vi "Start Call to results window.vi"(8 "Find Broadcast?":bool, 9 "Request VI Callers":refnum<vi>[](array[refnum]), 10 "Event":refnum<vi>) -> ()   [LabVIEW 2020, in "Panther Dashboard.lvlib"]
uses:
  Panther Dashboard.lvlib
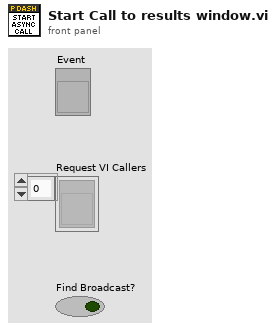
[diagram p1: front panel]
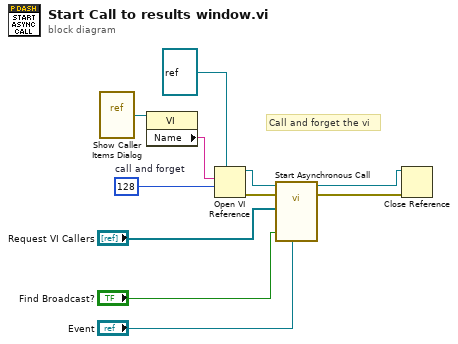
[diagram p0: block diagram]
diagram:
  w8 = 128  # call and forget
  # "Call and forget the vi"
  n1 = vi-ref "Show Caller Items Dialog.vi"() -> (w5:refnum<vi>)
  n2 = property class="VI"(reference=w5) -> ("Name"=w6:string)  [unwired: 1 in, 2 out]
  n3 = Open VI Reference(type specifier VI Refnum (for type only)=refnum<vi> refnum, vi path=w6, options=w8) -> (vi reference=w4:refnum<vi>, error out=w10:errorcluster)  [unwired: 3 in]
  n4 = call-by-ref "Start Asynchronous Call"(reference=w4, error in=w10, "Event"="Event", "Find Broadcast?"="Find Broadcast?", "Request VI Callers"="Request VI Callers") -> (reference out=w7:refnum<vi>, error out=w11:errorcluster)  [unwired: 9 in]
  n5 = Close Reference(reference=w7, error in (no error)=w11) -> ()  [unwired: 1 out]
